vi "cond FFT.vi"() -> ()   [LabVIEW 2016]
uses:
  <vilib>/Analysis/baseanly.llb/Mean (DBL).vi
  <vilib>/measure/maresamp.llb/Resample Pair of Arrays (single shot).vi
  <vilib>/measure/maspectr.llb/FFT Power Spectrum and PSD for 1 Chan.vi
  <vilib>/measure/NI_MAPro.lvlib
  <vilib>/Analysis/NI_AALBase.lvlib
panel:
  out "conductance":cluster{dbl[], dbl[]}(graph)
  out "Resampled data":waveform(dbl)(graph)={"t0"=timestamp(-3.552713678800501e-15 s since 1904-01-01), "dt"=0.05, "Y"=[]}
  out "FFT (1/um)":cluster{"f0":dbl, "df":dbl, "magnitude":dbl[]}(graph)={"f0"=0.0, "df"=0.055401662049861494, "magnitude"=[]}
  in  "t0":dbl format="%.2p"
  in  "dt":dbl=0.05 format="%.2p"
  in  "Cond intensity":dbl[][](graph)
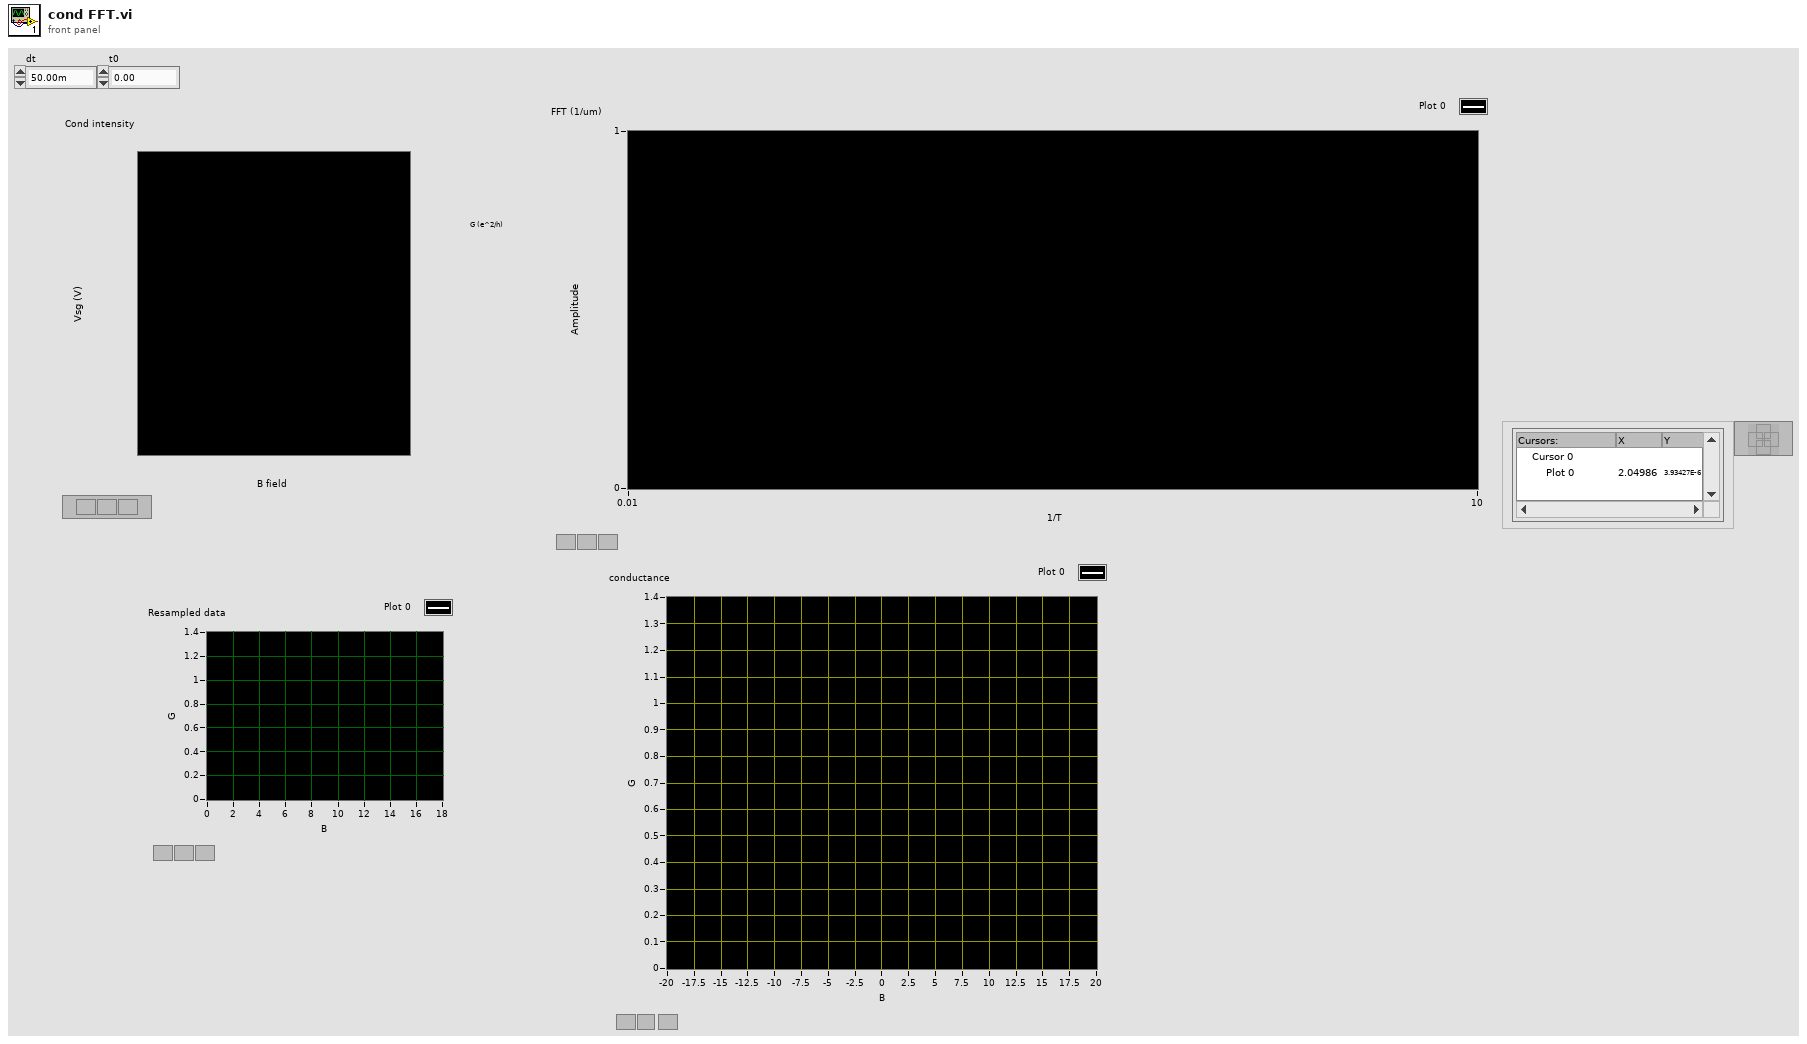
[diagram p1: front panel]
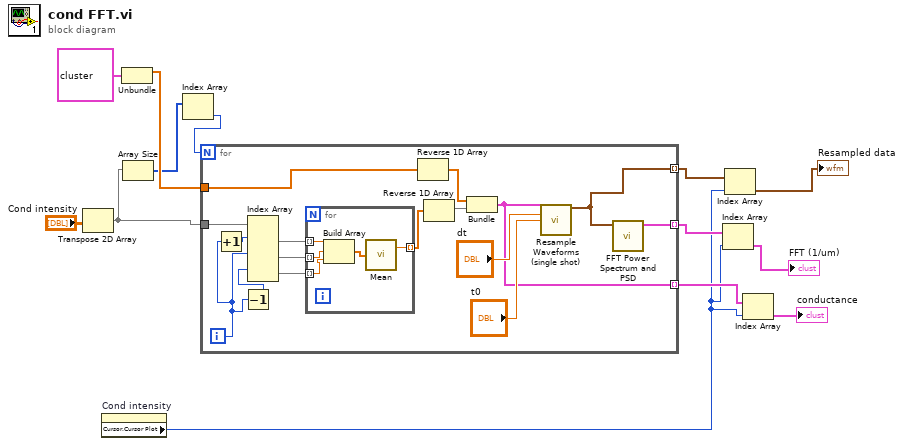
[diagram p0: block diagram]
diagram:
  n1 = Transpose 2D Array(2D array="Cond intensity") -> (transposed array=w3:dbl[][])
  n2 = property on="Cond intensity" class="IntGraph (strict)"() -> ("Cursor.Cursor Plot"=w5:i32)  [unwired: 2 in, 2 out]
  n3 = Unbundle(cluster{dbl[], dbl[]} {array[692 elements], array[692 elements]} ("horizontal line cut")) -> (w11:dbl[])  [unwired: 1 out]
  n4 = Array Size(array=w3) -> (size(s)=w2:i32[])
  n5 = Index Array(array=w2) -> (element=w1:i32)  [unwired: 1 in]
  n6 = for {
    N: w1 -> [_]
    tunnel: w3 -> [w21]
    tunnel: w11 -> [w24]
    tunnel: [w27] -> w10 mode=indexing
    tunnel: [w26] -> w9 mode=indexing
    tunnel: [w25] -> w6 mode=indexing
    i -> [w19]
    n7 = Increment(x=w19) -> (x+1=w20:i32)
    n8 = Decrement(x=w19) -> (x-1=w18:i32)
    n9 = Index Array(array=w21, index (row) #1=w20, index (row) #2=w19, index (row) #3=w18) -> (element #1=w17:dbl[], element #2=w16:dbl[], element #3=w15:dbl[])  [unwired: 3 in]
    n10 = for {
      tunnel: w17 -> [w34] mode=indexing
      tunnel: w16 -> [w33] mode=indexing
      tunnel: w15 -> [w32] mode=indexing
      tunnel: [w30] -> w14 mode=indexing
      n11 = Build Array(w34, w33, w32) -> (w31:dbl[])
      n12 = call-poly <vilib>:"Mean.vi"("X"=w31) -> ("mean"=w30:dbl)  [unwired: 1 out]
    }
    n13 = Reverse 1D Array(array=w24) -> (reversed array=w23:dbl[])
    n14 = Reverse 1D Array(array=w14) -> (reversed array=w22:dbl[])
    n15 = Bundle(w23, w22) -> (w25:cluster{dbl[], dbl[]})  [unwired: 1 in]
    n16 = call-poly <vilib>:"Resample Waveforms (single shot).vi"("XY-data in"=w25, "dt"="dt", "t0"="t0") -> ("resampled waveform out"=w26:waveform(dbl))  [unwired: 8 in, 4 out]
    n17 = call-poly <vilib>:"FFT Power Spectrum and PSD.vi"("time signal"=w26) -> ("Power Spectrum / PSD"=w27:cluster{"f0":dbl, "df":dbl, "magnitude":dbl[]})  [unwired: 7 in, 3 out]
  }
  n18 = Index Array(array=w10, index=w5) -> (element=→"FFT (1/um)":cluster{"f0":dbl, "df":dbl, "magnitude":dbl[]})
  n19 = Index Array(array=w9, index=w5) -> (element=→"Resampled data":waveform(dbl))
  n20 = Index Array(array=w6, index=w5) -> (element=→"conductance":cluster{dbl[], dbl[]})
